vi "PQfetchColumnNames.vi"(6 "error in":errorcluster, 8 "res":u64, 9 "conn":u64) -> (0 "error out":errorcluster, 1 "ColumnNames":string[](array[string]), 2 "res_out":u64, 3 "conn_out":u64)   [LabVIEW 2019, in "libpqutility64.lvlib"]
doc: "Fetch Column Names for Result.\nSee PostgreSQL c-lib doku for further information."
uses:
  libpqutility64.lvlib
  libpqlv64/libpqlv64.lvlib
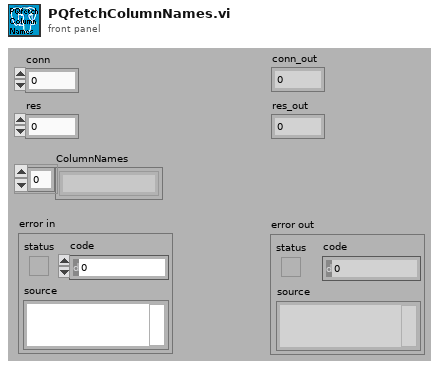
[diagram p1: front panel]
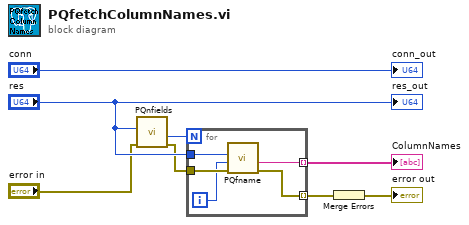
[diagram p0: block diagram]
diagram:
  n1 = call "PQnfields.vi"("error in (no error)"="error in", "res"="res") -> ("error out"=w3:errorcluster, "PQnFields"=w5:i64)  [unwired: 7 in, 1 out]
  n2 = for {
    N: w5 -> [_]
    tunnel: [w9] -> w8 mode=indexing
    tunnel: "res" -> [w10]
    tunnel: w3 -> [w13]
    tunnel: [w12] -> w1 mode=indexing
    i -> [w11]
    n3 = call "PQfname.vi"("error in (no error)"=w13, "cloumn_num"=w11, "res"=w10) -> ("error out"=w12:errorcluster, "ColumnName"=w9:string)  [unwired: 4 in, 1 out]
  }
  "ColumnNames" <- w8
  n4 = Merge Errors(w1) -> (→"error out":errorcluster)
  "res_out" <- "res"
  "conn_out" <- "conn"
